vi "Main.vi"() -> ()   [LabVIEW 2023]
uses:
  defs/Notification Definition.ctl
  defs/HTTP Queue Definition.ctl
  defs/Data.ctl
  <vilib>/userDefined/High Color/IMAQdx.ctl
panel:
  in  "Parametrs Confirmation":bool
  in  "Photo Period (ms)":u32=2000
  in  "RGB Camera Session":refnum<k21> caption="IMAQdx Session"
  in  "Stop":bool
  out "error out":errorcluster
  in  "Hyperspectral Camera Session":T1
  in  "Photo Save Directory":path
  # "Cameras Initialization"
  # "Steps:\n - start VI\n - setup initialization parameters\n - confirm parameters"
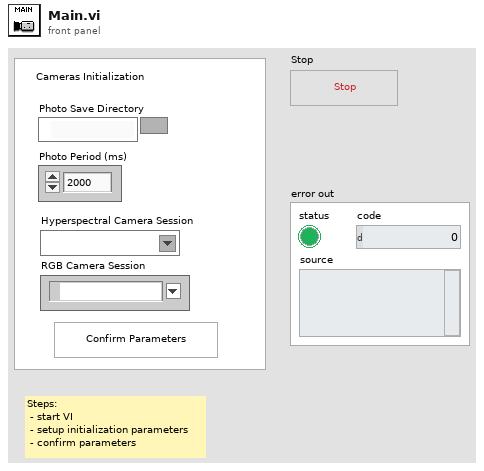
[diagram p1: front panel]
types:
  T1 = typedef "IMAQdx.ctl" = refnum<k21>
  T2 = typedef "Data.ctl" = cluster{"HTTP Queue":refnum<queue>, "Notifier":refnum<notifier>, "Photo Save Directory":path, "Photo Period (ms)":u32}
  T3 = typedef "HTTP Queue Definition.ctl" = cluster{"Message":string, "Photo Path":path}
  T4 = typedef "Notification Definition.ctl" = cluster{"Message":string}
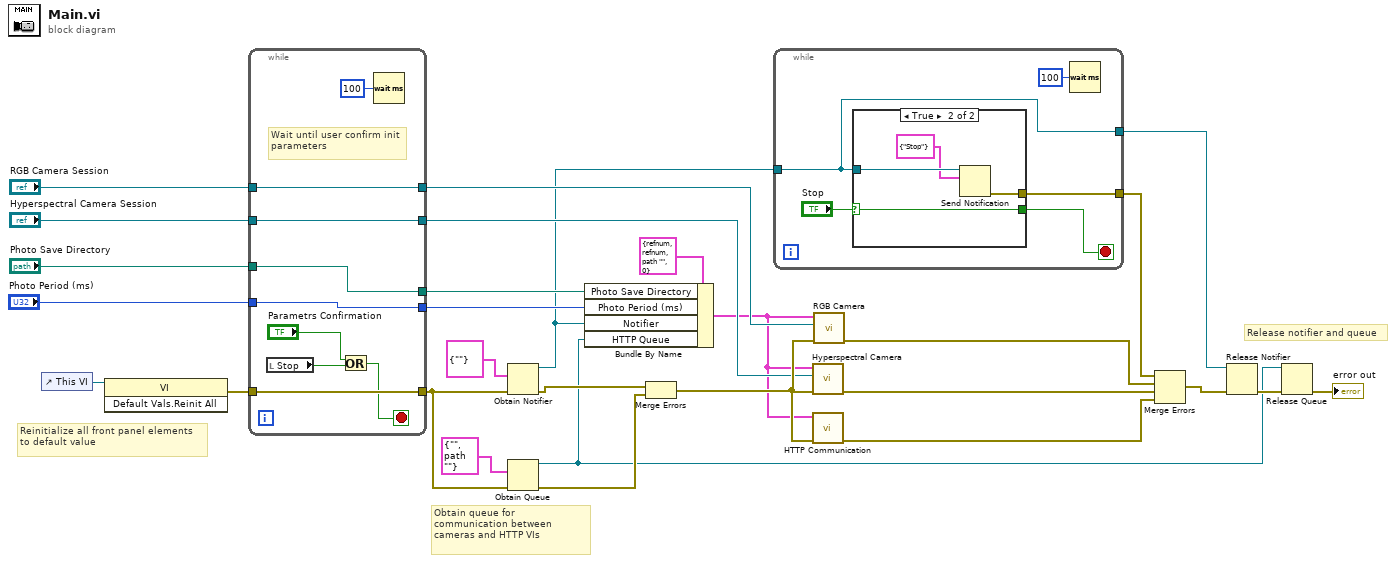
[diagram p0: block diagram]
diagram:
  # "Release notifier and queue"
  # "Obtain queue for communication between cameras and HTTP VIs"
  # "Reinitialize all front panel elements to default value"
  n1 = control-ref of="This VI"() -> (w24:refnum<vi>)
  n2 = invoke class="VI" method="Default Vals.Reinit All"(reference=w24) -> (error out=w15:errorcluster)  [unwired: 2 in, 2 out]
  n3 = while {
    tunnel: w15 -> [w37]
    tunnel: [w37] -> w14
    tunnel: "Photo Period (ms)" -> [w36]
    tunnel: "Photo Save Directory" -> [w35]
    tunnel: "Hyperspectral Camera Session" -> [w34]
    tunnel: "RGB Camera Session" -> [w33]
    tunnel: [w36] -> w4
    tunnel: [w35] -> w5
    tunnel: [w34] -> w9
    tunnel: [w33] -> w8
    stop <- w32 stop-if-true
    # "Wait until user confirm init parameters"
    n4 = local read "Stop"() -> (w31:bool)
    n5 = Or(x="Parametrs Confirmation", y=w31) -> (x .or. y?=w32:bool)
    n6 = Wait (ms)(milliseconds to wait=u32 100) -> ()  [unwired: 1 out]
  }
  n7 = Obtain Notifier(notification data type=T4 {"Message"=""} ("Event Handling Message"), error in (no error)=w14) -> (notifier out=w3:refnum<notifier>, error out=w20:errorcluster)  [unwired: 2 in, 1 out]
  n8 = Obtain Queue(element data type=T3 {"Message"="", "Photo Path"=path ""}, error in (no error)=w14) -> (queue out=w2:refnum<queue>, error out=w21:errorcluster)  [unwired: 3 in, 1 out]
  n9 = Bundle By Name(cluster=T2 {"HTTP Queue"=refnum, "Notifier"=refnum, "Photo Save Directory"=path "", "Photo Period (ms)"=0} ("Data"), "Photo Save Directory"=w5, "Photo Period (ms)"=w4, "Notifier"=w3, "HTTP Queue"=w2) -> (w6:T2)
  n10 = Merge Errors(w20, w21) -> (w19:errorcluster)
  n11 = while {
    tunnel: w3 -> [w38]
    tunnel: [w42] -> w23
    tunnel: [w38] -> w1
    stop <- w40 stop-if-true
    n12 = case shown="True" "Stop" {
      selector: "Stop" -> [_ w43]
      tunnel: w38 -> [_ w46]
      tunnel: [_ w45] -> w42
      tunnel: [_ w43] -> w40
      frame False {
      }
      frame True {
        n13 = Send Notification(notification=T4 {"Message"="Stop"}, notifier=w46) -> (error out=w45:errorcluster)  [unwired: 1 in, 1 out]
      }
    }
    n14 = Wait (ms)(milliseconds to wait=u32 100) -> ()  [unwired: 1 out]
  }
  n15 = call "Hyperspectral Camera.vi"("error in"=w19, "Hyperspectral Camera Session"=w9, "Data"=w6) -> ("error out"=w27:errorcluster)  [unwired: 8 in]
  n16 = call "HTTP Communication.vi"("error in"=w19, "Data"=w6) -> ("error out"=w18:errorcluster)  [unwired: 9 in]
  n17 = call "RGB Camera.vi"("error in"=w19, "RGB Camera Session"=w8, "Data"=w6) -> ("error out"=w26:errorcluster)  [unwired: 8 in]
  n18 = Merge Errors(w23, w26, w27, w18) -> (w25:errorcluster)
  n19 = Release Notifier(notifier=w1, error in (no error)=w25) -> (error out=w17:errorcluster)  [unwired: 1 in, 2 out]
  n20 = Release Queue(queue=w2, error in (no error)=w17) -> (error out=→"error out":errorcluster)  [unwired: 1 in, 2 out]
